vi "ejer5.vi"() -> ()   [LabVIEW 2014]
panel:
  in  "Pestañas":T1(tab)
  in  "Frecuencia":dbl(knob) scale=0.0..100.0
  in  "Amplitud":dbl(knob) scale=0.0..100.0
  out "Waveform Chart":dynamicdata(graph)
  out "Aleatorios":dbl[](array[numeric])
  out "Cantidad de números generados":i32
  out "Primos":dbl[](array[numeric])
  out "Cantidad de números primos":i32
  out "Pares":dbl[](array[numeric])
  out "Impares":dbl[](array[numeric])
  out "Cantidad de números pares":i32
  out "Cantidad de números impares":i32
  out "Mensaje Final":string
  in  "Número del mes de nacimiento":dbl
  in  "Año de nacimiento":dbl
  in  "Nombres y Apellidos":string
  out "Matriz Trapuesta":dbl[][](array[numeric])
  out "Matriz Original":dbl[][](array[numeric])
  out "Máximos":dbl[](array[numeric])
  out "Mínimos":dbl[](array[numeric])
  in  "STOP":bool
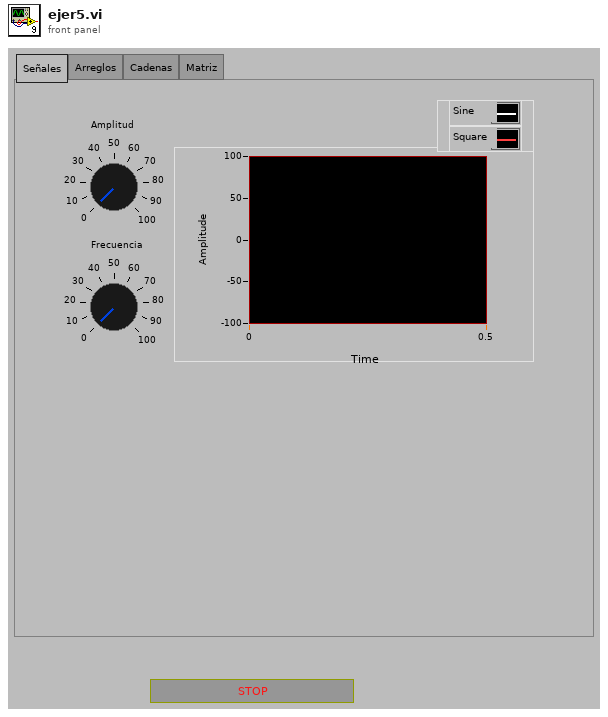
[diagram p1: front panel]
types:
  T1 = enum32{"Señales", "Arreglos", "Cadenas", "Matriz"}
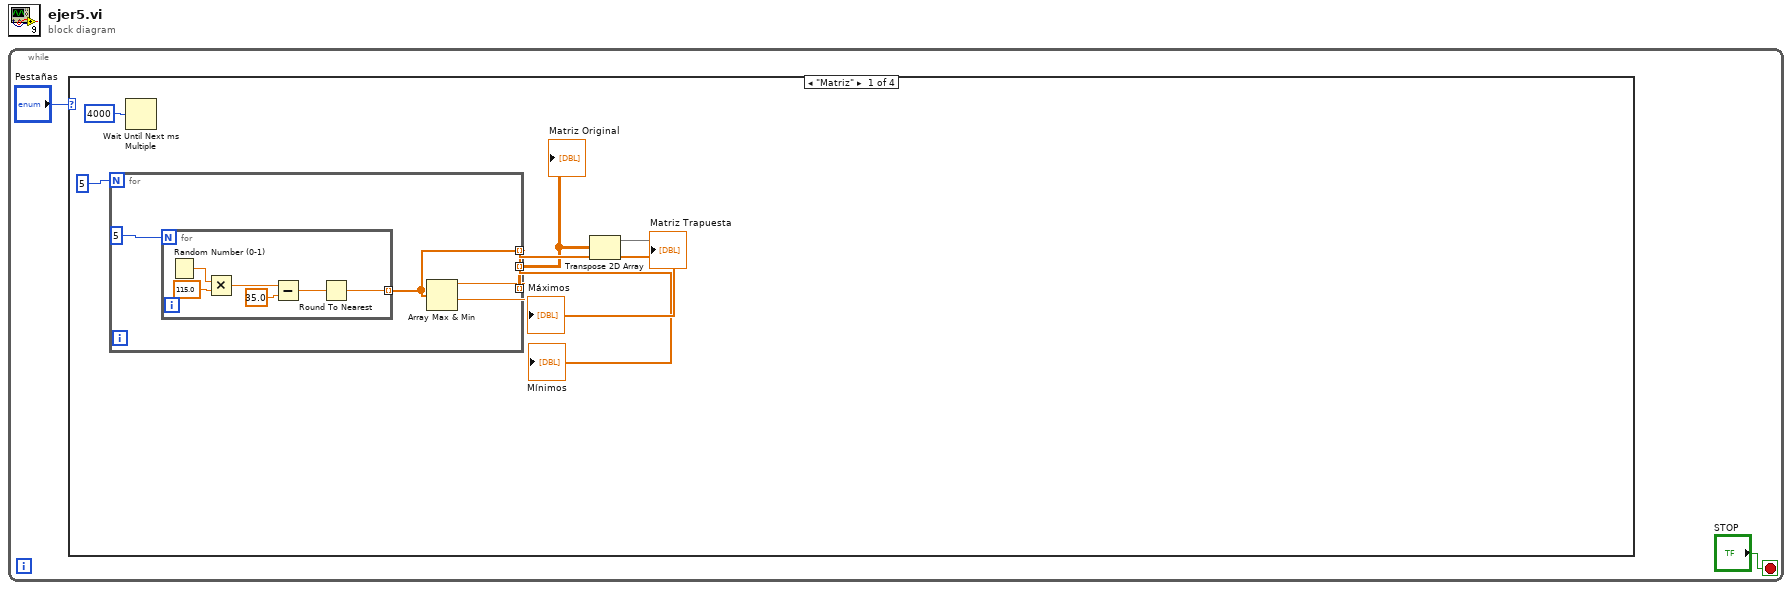
[diagram p0: block diagram]
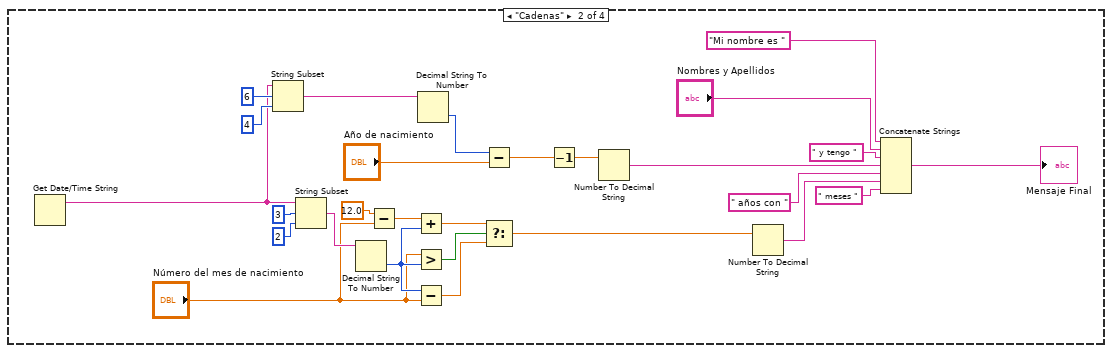
[diagram p2: hidden frame]
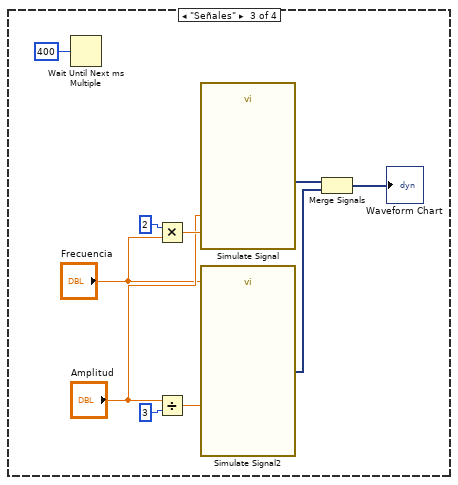
[diagram p3: hidden frame]
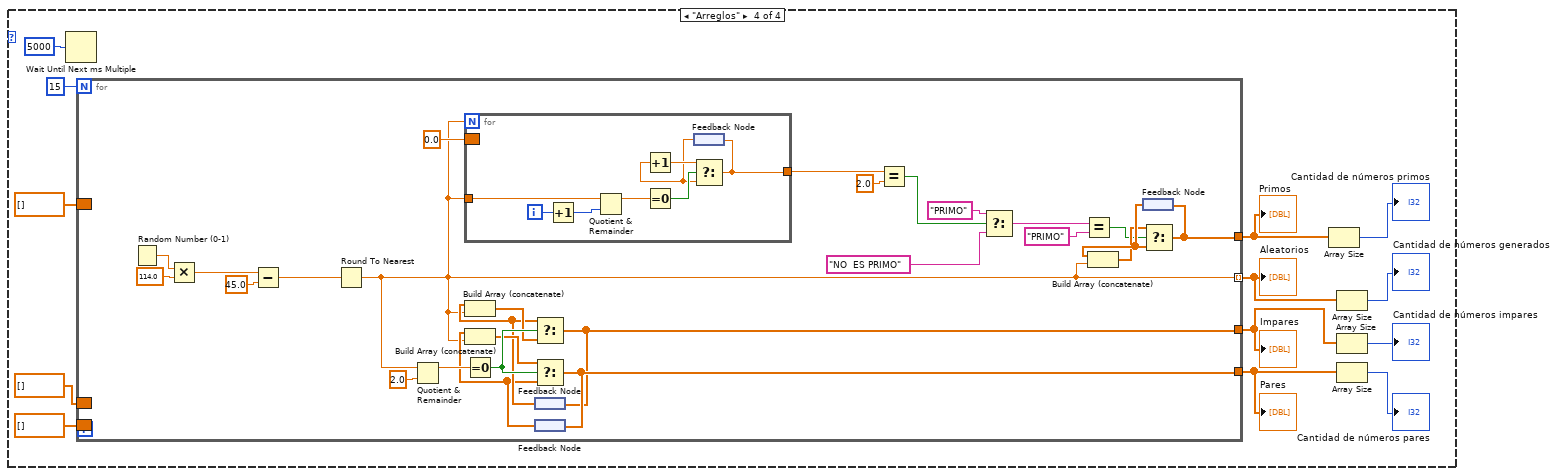
[diagram p4: hidden frame]
diagram:
  n1 = while {
    stop <- "STOP" stop-if-true
    n2 = case shown="\"Matriz\"" "Pestañas" {
      frame "Matriz" {
        n3 = for {
          N: 5 -> [_]
          tunnel: [w11] -> w3 mode=indexing
          tunnel: [w10] -> w5 mode=indexing
          tunnel: [w9] -> w4 mode=indexing
          n4 = for {
            N: 5 -> [_]
            tunnel: [w14] -> w11 mode=indexing
            n5 = Random Number (0-1)() -> (number: 0 to 1=w18:dbl)
            n6 = Multiply(x=w18, y=115.0) -> (x*y=w13:dbl)
            n7 = Subtract(x=w13, y=35.0) -> (x-y=w15:dbl)
            n8 = Round To Nearest(number=w15) -> (nearest integer value=w14:dbl)
          }
          n9 = Array Max & Min(array=w11) -> (max value=w10:dbl, min value=w9:dbl)  [unwired: 2 out]
        }
        "Matriz Original" <- w3
        "Máximos" <- w5
        "Mínimos" <- w4
        n10 = Wait Until Next ms Multiple(millisecond multiple=u32 4000) -> ()  [unwired: 1 out]
        n11 = Transpose 2D Array(2D array=w3) -> (transposed array=→"Matriz Trapuesta":dbl[][])
      }
      frame "Cadenas" {
        n12 = Get Date/Time String() -> (date string=w22:string)  [unwired: 3 in, 1 out]
        n13 = String Subset(string=w22, offset (0)=6, length (rest)=4 ("length (rest)")) -> (substring=w37:string)
        n14 = String Subset(string=w22, offset (0)=3, length (rest)=2 ("length (rest)")) -> (substring=w40:string)
        n15 = Decimal String To Number(string=w40) -> (number=w31:i32)  [unwired: 2 in, 1 out]
        n16 = Subtract(x=12.0, y="Número del mes de nacimiento") -> (x-y=w32:dbl)
        n17 = Add(x=w32, y=w31) -> (x+y=w23:dbl)
        n18 = Greater?(x="Número del mes de nacimiento", y=w31) -> (0:w34:bool)
        n19 = Subtract(x=w31, y="Número del mes de nacimiento") -> (x-y=w30:dbl)
        n20 = Decimal String To Number(string=w37) -> (number=w25:i32)  [unwired: 2 in, 1 out]
        n21 = Subtract(x=w25, y="Año de nacimiento") -> (x-y=w21:dbl)
        n22 = Select(t=w23, s=w34, f=w30) -> (s? t:f=w29:dbl)
        n23 = Decrement(x=w21) -> (x-1=w20:dbl)
        n24 = Number To Decimal String(number=w20) -> (decimal integer string=w36:string)  [unwired: 1 in]
        n25 = Number To Decimal String(number=w29) -> (decimal integer string=w28:string)  [unwired: 1 in]
        n26 = Concatenate Strings "Concatenate Strings"("Mi nombre es " ("string"), "Nombres y Apellidos", " y tengo " ("string"), w36, " años con " ("string"), w28, " meses " ("string")) -> (→"Mensaje Final":string)
      }
      frame "Señales" {
        n27 = Wait Until Next ms Multiple(millisecond multiple=u32 400) -> ()  [unwired: 1 out]
        n28 = Multiply(x=2, y="Frecuencia") -> (x*y=w51:dbl)
        n29 = Divide(x="Amplitud", y=3) -> (x/y=w47:dbl)
        n30 = call "Simulate Signal"("Frequency"=w51, "Amplitude"="Amplitud") -> ("Sine"=w52:dynamicdata)  [unwired: 12 in, 1 out]
        n31 = call "Simulate Signal2"("Frequency"="Frecuencia", "Amplitude"=w47) -> ("Square"=w55:dynamicdata)  [unwired: 12 in, 1 out]
        n32 = Merge Signals(w52, w55) -> (→"Waveform Chart":dynamicdata)
      }
      frame "Arreglos" {
        n33 = Wait Until Next ms Multiple(millisecond multiple=5000) -> ()  [unwired: 1 out]
        n34 = for {
          N: 15 -> [_]
          tunnel: [w69] -> w57 mode=indexing
          tunnel: [w89] -> w65
          tunnel: [w87] -> w62
          tunnel: [w83] -> w60
          border: dbl[] [] -> [_]
          border: dbl[] [] -> [_]
          border: dbl[] [] -> [_]
          n35 = Random Number (0-1)() -> (number: 0 to 1=w95:dbl)
          n36 = Multiply(x=w95, y=114.0) -> (x*y=w93:dbl)
          n37 = Subtract(x=w93, y=45.0 ("x*y")) -> (x-y=w88:dbl)
          n38 = Round To Nearest(number=w88) -> (nearest integer value=w69:dbl)
          n39 = Quotient & Remainder(x=w69, y=2.0) -> (x-y*floor(x/y)=w85:dbl)  [unwired: 1 out]
          n40 = for {
            N: w69 -> [_]
            tunnel: w69 -> [w102]
            tunnel: [w96] -> w76
            border: 0.0 -> [_]
            i -> [w103]
            n41 = Increment(x=w103) -> (x+1=w101:i32)
            n42 = Quotient & Remainder(x=w102, y=w101) -> (x-y*floor(x/y)=w100:dbl)  [unwired: 1 out]
            n43 = Equal To 0?(x=w100) -> (x = 0?=w99:bool)
            n44 = feedback #1() -> (w97:dbl)
            n45 = Increment(x=w97) -> (x+1=w98:dbl)
            n46 = Select(t=w98, s=w99, f=w97) -> (s? t:f=w96:dbl)
            n47 = feedback-in #1(w96) -> ()
          }
          n48 = Equal To 0?(x=w85) -> (x = 0?=w86:bool)
          n49 = feedback #2() -> (w79:dbl[])
          n50 = Build Array (concatenate)(w79, w69) -> (w84:dbl[])
          n51 = Select(t=w79, s=w86, f=w84) -> (s? t:f=w83:dbl[])
          n52 = feedback-in #2(w83) -> ()
          n53 = feedback #3() -> (w78:dbl[])
          n54 = Build Array (concatenate)(w78, w69) -> (w81:dbl[])
          n55 = Select(t=w81, s=w86, f=w78) -> (s? t:f=w87:dbl[])
          n56 = feedback-in #3(w87) -> ()
          n57 = Equal?(x=w76, y=2.0) -> (x = y?=w74:bool)
          n58 = Select(t="PRIMO", s=w74, f="NO  ES PRIMO") -> (s? t:f=w70:string)
          n59 = Equal?(x=w70, y="PRIMO") -> (x = y?=w80:bool)
          n60 = feedback #4() -> (w90:dbl[])
          n61 = Build Array (concatenate)(w90, w69) -> (w82:dbl[])
          n62 = Select(t=w82, s=w80, f=w90) -> (s? t:f=w89:dbl[])
          n63 = feedback-in #4(w89) -> ()
        }
        "Aleatorios" <- w57
        "Primos" <- w65
        "Pares" <- w62
        "Impares" <- w60
        n64 = Array Size(array=w65) -> (size(s)=→"Cantidad de números primos":i32)
        n65 = Array Size(array=w57) -> (size(s)=→"Cantidad de números generados":i32)
        n66 = Array Size(array=w60) -> (size(s)=→"Cantidad de números impares":i32)
        n67 = Array Size(array=w62) -> (size(s)=→"Cantidad de números pares":i32)
      }
    }
  }
